vi "Get Laser Status.vi"() -> ()   [LabVIEW 2022 SP3]
panel:
  out "error out":errorcluster
  out "GetMaxPower 2":dbl
  out "GetMaxPower":dbl
  out "Numeric":i32
  out "GetOutputPower 2":dbl
  out "GetOutputPower":dbl
  in  "stop":bool
  out "Status 2":string[](array[string])
  in  "BSALaserCtrl.IBSALaser 2":refnum<k7>
  out "Status":string[](array[string])
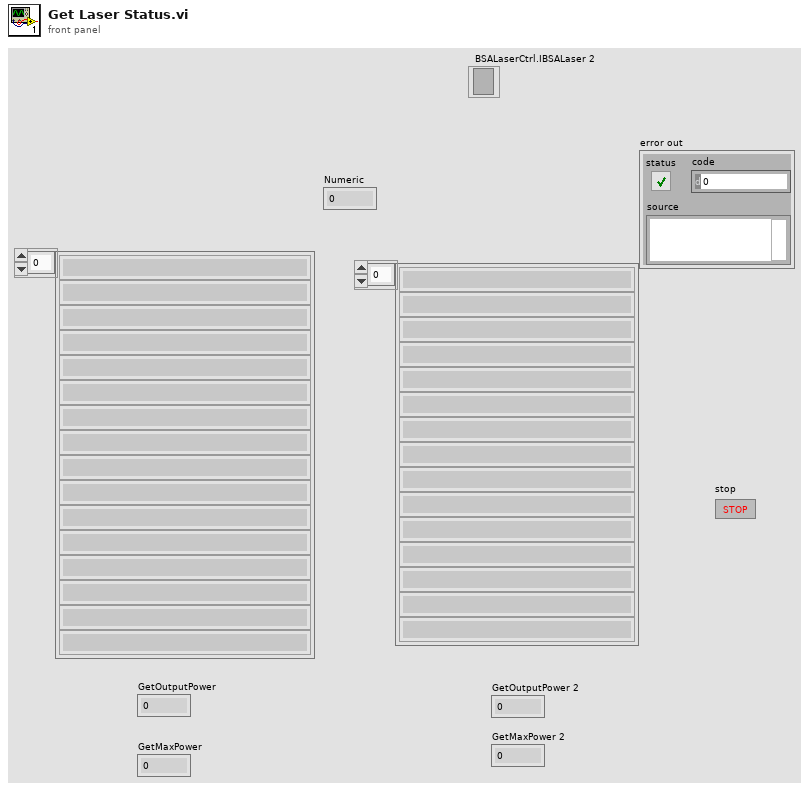
[diagram p1: front panel]
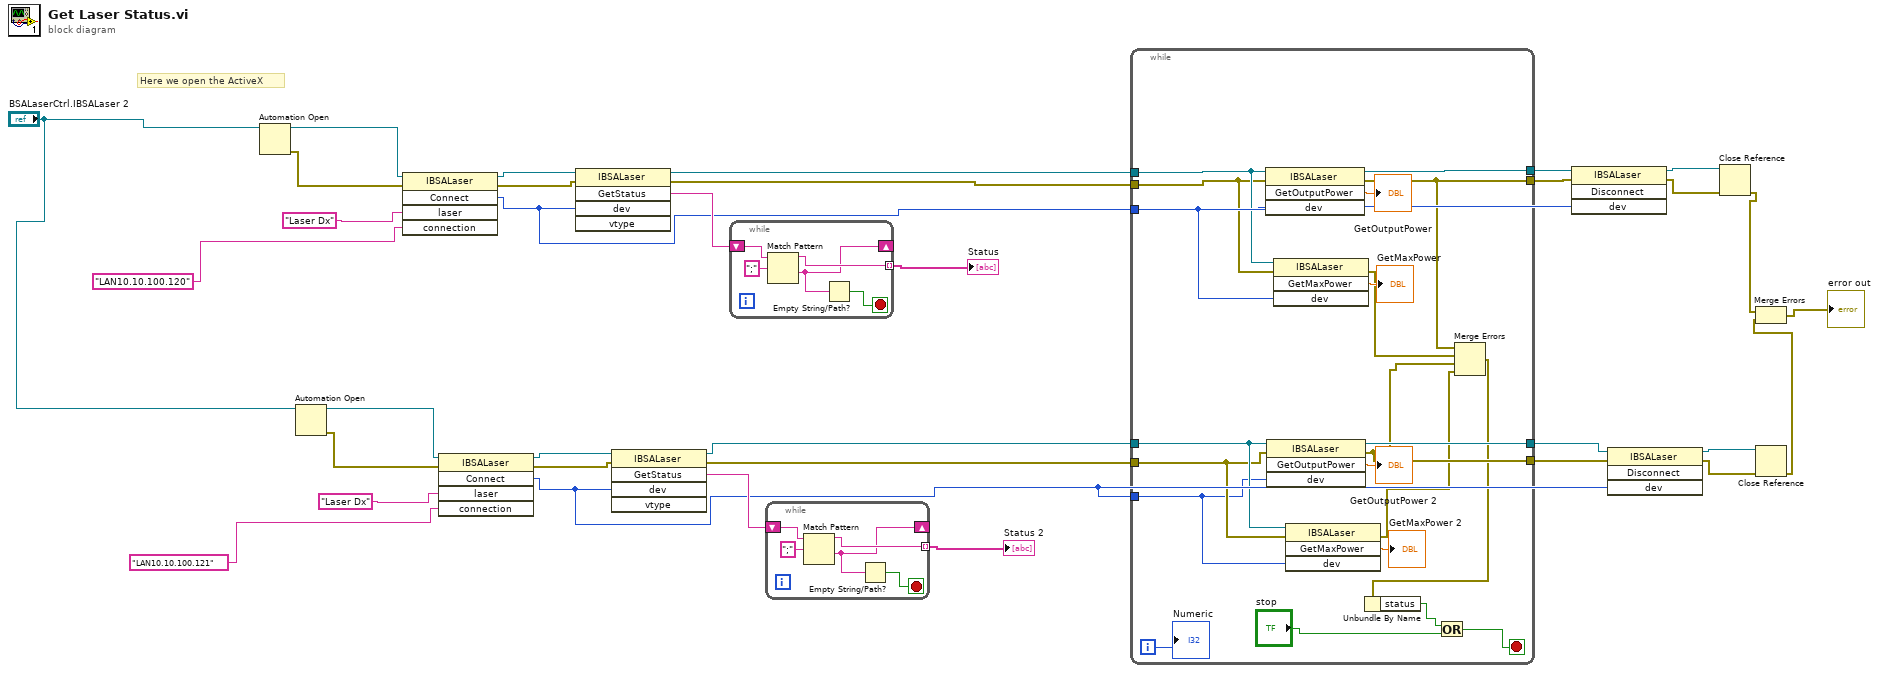
[diagram p0: block diagram]
diagram:
  # "Here we open the ActiveX"
  n1 = Automation Open(Automation Refnum="BSALaserCtrl.IBSALaser 2") -> (Automation Refnum=w28:refnum<k7>, error out=w27:errorcluster)  [unwired: 3 in]
  n2 = Automation Open(Automation Refnum="BSALaserCtrl.IBSALaser 2") -> (Automation Refnum=w21:refnum<k7>, error out=w22:errorcluster)  [unwired: 3 in]
  n3 = invoke class="IBSALaser" method="Connect"(reference=w28, error in=w27, "laser"="Laser Dx", "connection"="LAN10.10.100.120") -> (reference out=w30:refnum<k7>, error out=w29:errorcluster, "Connect"=w12:i32)  [unwired: 1 in, 2 out]
  n4 = invoke class="IBSALaser" method="Connect"(reference=w21, error in=w22, "laser"="Laser Dx", "connection"="LAN10.10.100.121") -> (reference out=w19:refnum<k7>, error out=w20:errorcluster, "Connect"=w13:i32)  [unwired: 1 in, 2 out]
  n5 = invoke class="IBSALaser" method="GetStatus"(reference=w30, error in=w29, "dev"=w12) -> (reference out=w11:refnum<k7>, error out=w10:errorcluster, "GetStatus"=w31:string)  [unwired: 2 in, 2 out]
  n6 = invoke class="IBSALaser" method="GetStatus"(reference=w19, error in=w20, "dev"=w13) -> (reference out=w7:refnum<k7>, error out=w6:errorcluster, "GetStatus"=w18:string)  [unwired: 2 in, 2 out]
  n7 = while {
    shift-right: [w35] -> _
    shift-left: w31 -> [w38]
    tunnel: [w37] -> w32 mode=indexing
    stop <- w36 stop-if-true
    n8 = Match Pattern(string=w38, regular expression=";") -> (before substring=w37:string, after substring=w35:string)  [unwired: 1 in, 2 out]
    n9 = Empty String/Path?(string/path=w35) -> (empty?=w36:bool)
  }
  "Status" <- w32
  n10 = while {
    shift-right: [w40] -> _
    shift-left: w18 -> [w43]
    tunnel: [w42] -> w17 mode=indexing
    stop <- w41 stop-if-true
    n11 = Match Pattern(string=w43, regular expression=";") -> (before substring=w42:string, after substring=w40:string)  [unwired: 1 in, 2 out]
    n12 = Empty String/Path?(string/path=w40) -> (empty?=w41:bool)
  }
  "Status 2" <- w17
  n13 = while {
    tunnel: w13 -> [w53]
    tunnel: w12 -> [w58]
    tunnel: w11 -> [w60]
    tunnel: w10 -> [w59]
    tunnel: [w65] -> w9
    tunnel: [w52] -> w8
    tunnel: w7 -> [w55]
    tunnel: w6 -> [w54]
    tunnel: [w64] -> w5
    tunnel: [w50] -> w4
    i -> [w61]
    stop <- w45 stop-if-true
    n14 = invoke class="IBSALaser" method="GetOutputPower"(reference=w60, error in=w59, "dev"=w58) -> (reference out=w65:refnum<k7>, error out=w52:errorcluster, "GetOutputPower"=→"GetOutputPower":dbl)  [unwired: 1 in, 1 out]
    n15 = invoke class="IBSALaser" method="GetOutputPower"(reference=w55, error in=w54, "dev"=w53) -> (reference out=w64:refnum<k7>, error out=w50:errorcluster, "GetOutputPower"=→"GetOutputPower 2":dbl)  [unwired: 1 in, 1 out]
    n16 = invoke class="IBSALaser" method="GetMaxPower"(reference=w60, error in=w59, "dev"=w58) -> (error out=w51:errorcluster, "GetMaxPower"=→"GetMaxPower":dbl)  [unwired: 1 in, 2 out]
    n17 = invoke class="IBSALaser" method="GetMaxPower"(reference=w55, error in=w54, "dev"=w53) -> (error out=w49:errorcluster, "GetMaxPower"=→"GetMaxPower 2":dbl)  [unwired: 1 in, 2 out]
    n18 = Merge Errors(w52, w51, w50, w49) -> (w48:errorcluster)
    n19 = Unbundle By Name(w48) -> ("status"=w47:bool)
    n20 = Or(x=w47, y="stop") -> (x .or. y?=w45:bool)
    "Numeric" <- w61
  }
  n21 = invoke class="IBSALaser" method="Disconnect"(reference=w9, error in=w8, "dev"=w12) -> (reference out=w26:refnum<k7>, error out=w25:errorcluster)  [unwired: 1 in, 2 out]
  n22 = invoke class="IBSALaser" method="Disconnect"(reference=w5, error in=w4, "dev"=w13) -> (reference out=w23:refnum<k7>, error out=w24:errorcluster)  [unwired: 1 in, 2 out]
  n23 = Close Reference(reference=w26, error in (no error)=w25) -> (error out=w3:errorcluster)
  n24 = Close Reference(reference=w23, error in (no error)=w24) -> (error out=w2:errorcluster)
  n25 = Merge Errors(w3, w2) -> (→"error out":errorcluster)
